vi "DrivePID.vi"(0 "LeftDriveRefNum":string="My Encoder RefNum", 1 "RightDriveRefNum":string="My Encoder RefNum", 2 "SetpointLeft":dbl format="%.2f", 3 "SetpointRight":dbl format="%.2f", 4 "PID gains":T1={"proportional gain (Kc)"=0.5, "integral time (Ti, min)"=0.01, "derivative time (Td, min)"=0.0} {"derivative time (Td, min)" format="%.3f"; "integral time (Ti, min)" format="%.3f"; "proportional gain (Kc)" format="%.3f"}) -> (8 "Left Motor Output":dbl format="%.2f", 9 "Right Motor Output":dbl format="%.2f", 10 "Done":bool)   [LabVIEW 2014]
uses:
  <vilib>/addons/control/pid/pid.llb/PID (DBL).vi
  <vilib>/addons/control/pid/NI_PID_pid.lvlib
panel:
  out "Right Chart":dbl(graph)
  out "Left Chart":dbl(graph)
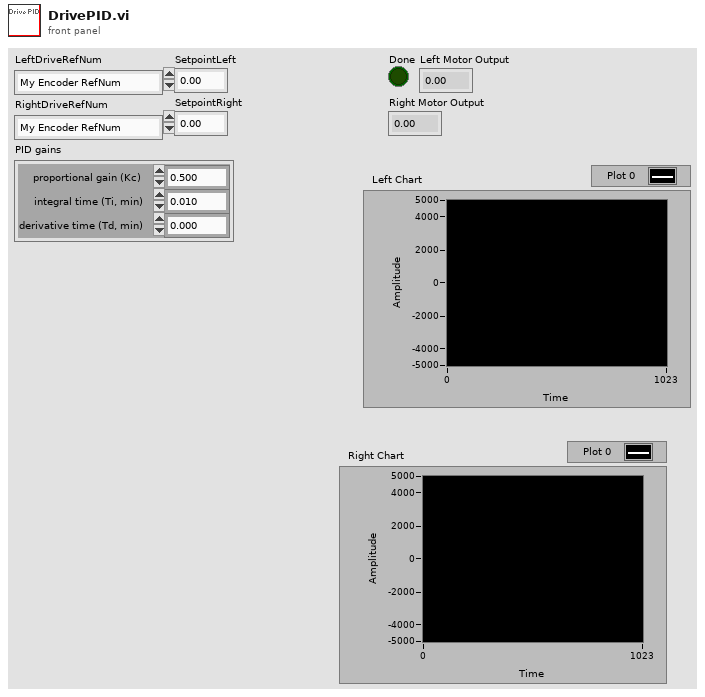
[diagram p1: front panel]
types:
  T1 = cluster{"proportional gain (Kc)":dbl, "integral time (Ti, min)":dbl, "derivative time (Td, min)":dbl}
  T2 = typedef "WPI_EncoderDevRef.ctl" = cluster{"DevStatus":errorcluster, "EncoderIndex":T3, "CounterIndex":T4, "DistancePerCount":dbl, "Decoding Type":T5}
  T3 = typedef "FPGA_EncoderIdx.ctl" = enum8{"Enc 0", "Enc 1", "Enc 2", "Enc 3", "Enc 4", "Enc 5", "Enc 6", "Enc 7", "Invalid"}
  T4 = typedef "FPGA_CounterCtrSystemIndex.ctl" = enum8{"Ctr 0", "Ctr 1", "Ctr 2", "Ctr 3", "Ctr 4", "Ctr 5", "Ctr 6", "Ctr 7", "Invalid"}
  T5 = typedef "WPI_EncoderType.ctl" = enum16{"1x", "2x", "4x"}
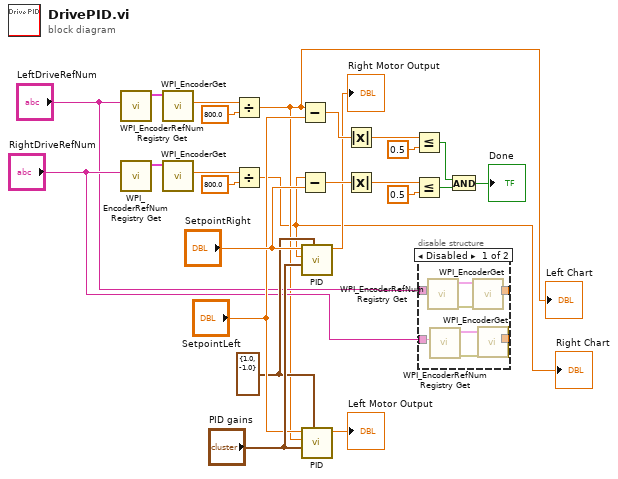
[diagram p0: block diagram]
diagram:
  w5 = cluster{"output high":dbl, "output low":dbl} {"output high"=1.0, "output low"=-1.0} ("output range")
  n1 = call <vilib>:"WPI_EncoderRefNum Registry Get.vi"("refnum name"="LeftDriveRefNum") -> ("EncoderDevRef"=w24:T2)  [unwired: 9 in, 1 out]
  n2 = call <vilib>:"WPI_EncoderRefNum Registry Get.vi"("refnum name"="RightDriveRefNum") -> ("EncoderDevRef"=w25:T2)  [unwired: 9 in, 1 out]
  n3 = call <vilib>:"WPI_EncoderGet.vi"("EncoderDevRef"=w24) -> ("Distance"=w22:dbl)  [unwired: 5 in, 5 out]
  n4 = call <vilib>:"WPI_EncoderGet.vi"("EncoderDevRef"=w25) -> ("Distance"=w20:dbl)  [unwired: 5 in, 5 out]
  n5 = Divide(x=w22, y=800.0) -> (x/y=w2:dbl)
  "Left Chart" <- w2
  n6 = Divide(x=w20, y=800.0) -> (x/y=w1:dbl)
  "Right Chart" <- w1
  n7 = Subtract(x=w2, y="SetpointLeft") -> (x-y=w14:dbl)
  n8 = Subtract(x=w1, y="SetpointRight") -> (x-y=w18:dbl)
  n9 = call-poly <vilib>:"PID.vi"("output range"=w5, "PID gains"="PID gains", "process variable"=w1, "setpoint"="SetpointRight") -> ("output"=→"Right Motor Output":dbl)  [unwired: 6 in, 1 out]
  n10 = call-poly <vilib>:"PID.vi"("output range"=w5, "PID gains"="PID gains", "process variable"=w2, "setpoint"="SetpointLeft") -> ("output"=→"Left Motor Output":dbl)  [unwired: 6 in, 1 out]
  n11 = Absolute Value(x=w14) -> (abs(x)=w13:dbl)
  n12 = Absolute Value(x=w18) -> (abs(x)=w17:dbl)
  n13 = Less Or Equal?(x=w13, y=0.5) -> (x <= y?=w11:bool)
  n14 = Less Or Equal?(x=w17, y=0.5) -> (x <= y?=w15:bool)
  n15 = disable-structure shown="Disabled" {
    disable-tunnel: [w29 _] -> _
    disable-tunnel: [w28 _] -> _
    disable-tunnel: "RightDriveRefNum" -> [w27 _]
    disable-tunnel: "LeftDriveRefNum" -> [w26 _]
    frame Disabled {
      n16 = call <vilib>:"WPI_EncoderRefNum Registry Get.vi"("refnum name"=w26) -> ("error out"=w33:errorcluster, "EncoderDevRef"=w32:T2)  [unwired: 9 in]
      n17 = call <vilib>:"WPI_EncoderRefNum Registry Get.vi"("refnum name"=w27) -> ("error out"=w31:errorcluster, "EncoderDevRef"=w30:T2)  [unwired: 9 in]
      n18 = call <vilib>:"WPI_EncoderGet.vi"("error in (no error)"=w33, "EncoderDevRef"=w32) -> ("Distance"=w29:dbl)  [unwired: 4 in, 5 out]
      n19 = call <vilib>:"WPI_EncoderGet.vi"("error in (no error)"=w31, "EncoderDevRef"=w30) -> ("Distance"=w28:dbl)  [unwired: 4 in, 5 out]
    }
    frame Enabled {
    }
  }
  n20 = And(x=w11, y=w15) -> (x .and. y?=→"Done":bool)
